vi "New ThingeverseIO Descriptor.vi"(11 "ThingiverseIO Descriptor":T2) -> (3 "Descriptor":string)   [LabVIEW 2015]
uses:
  ThingiverseIO Descriptor.ctl
  ThingerseIO Type.ctl
panel:
  in  "ThingerseIO Type":T1
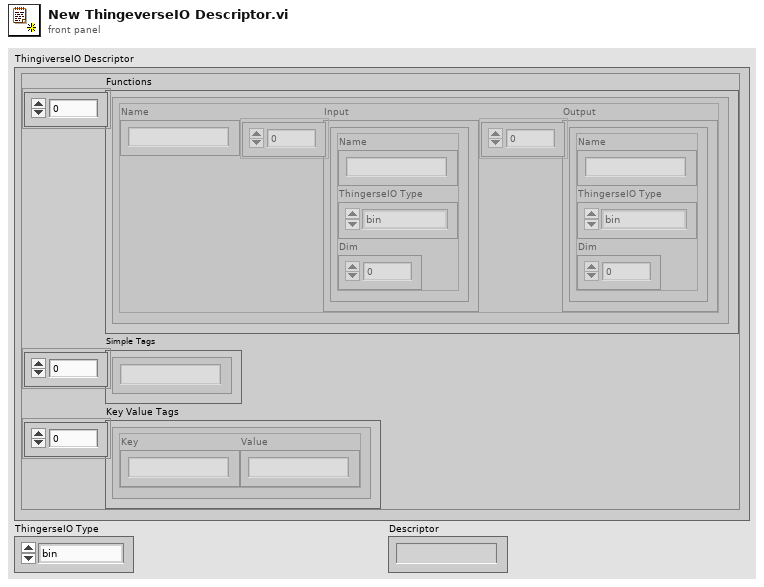
[diagram p1: front panel]
types:
  T1 = typedef "ThingerseIO Type.ctl" = enum16{"bin", "string", "Int", "float", "bool"}
  T2 = typedef "ThingiverseIO Descriptor.ctl" = cluster{"Functions":cluster{"Name":string, "Input":cluster{"Name":string, "ThingerseIO Type":T1, "Dim":u32}[], "Output":cluster{"Name":string, "ThingerseIO Type":T1, "Dim":u32}[]}[], "Simple Tags":string[], "Key Value Tags":cluster{"Key":string, "Value":string}[]}
  T3 = cluster{"Name":string, "Input":cluster{"Name":string, "ThingerseIO Type":T1, "Dim":u32}[], "Output":cluster{"Name":string, "ThingerseIO Type":T1, "Dim":u32}[]}[]
  T4 = cluster{"Name":string, "ThingerseIO Type":T1, "Dim":u32}[]
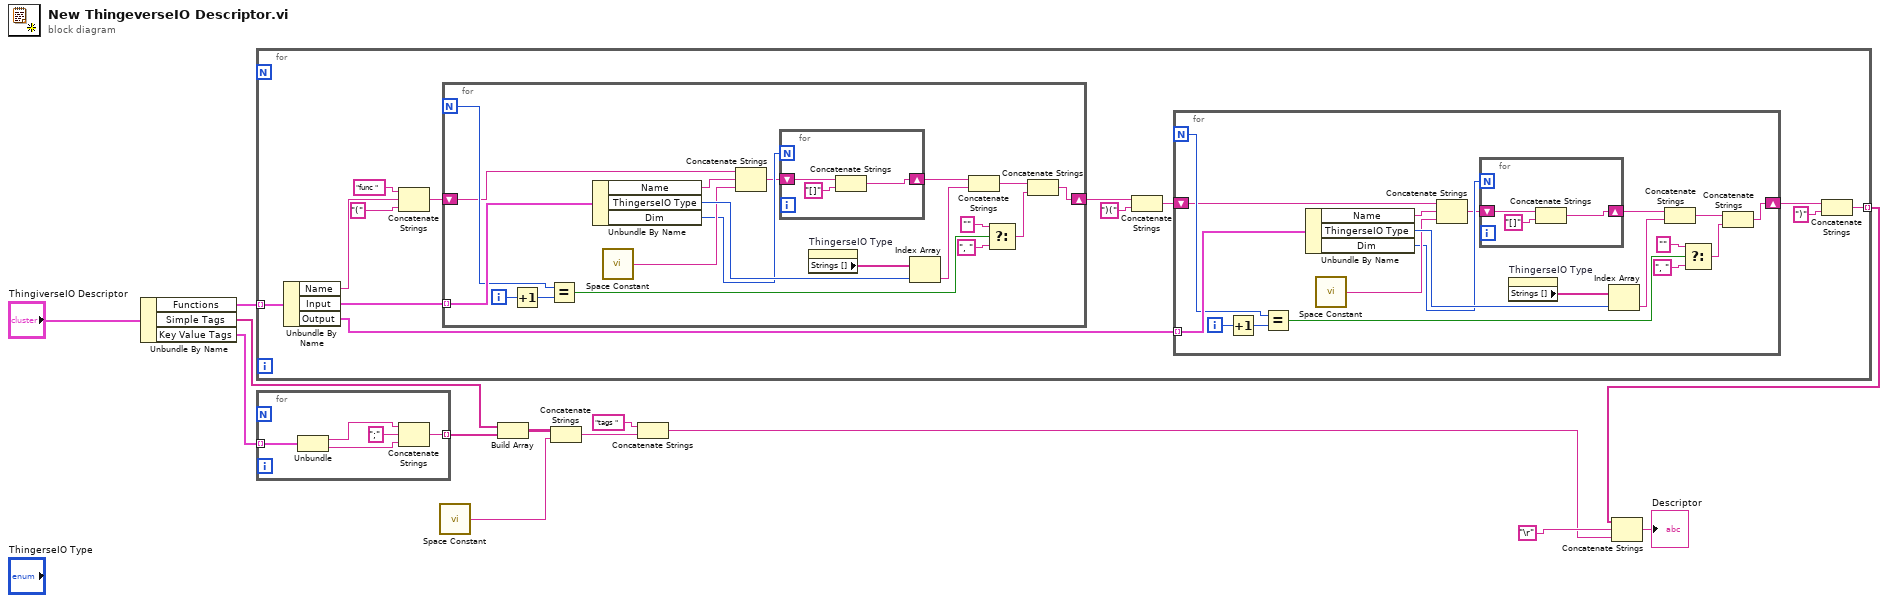
[diagram p0: block diagram]
diagram:
  n1 = Unbundle By Name("ThingiverseIO Descriptor") -> ("Functions"=w12:T3, "Simple Tags"=w10:string[], "Key Value Tags"=w11:cluster{"Key":string, "Value":string}[])
  n2 = for {
    tunnel: w12 -> [w25] mode=indexing
    tunnel: [w14] -> w4 mode=indexing
    n3 = Unbundle By Name(w25) -> ("Name"=w24:string, "Input"=w22:T4, "Output"=w18:T4)
    n4 = Concatenate Strings("func " ("string"), w24, "(" ("string")) -> (w21:string)
    n5 = for {
      N -> [w56]
      tunnel: w22 -> [w67] mode=indexing
      shift-right: [w49] -> w20
      shift-left: w21 -> [w50]
      i -> [w58]
      n6 = Increment(x=w58) -> (x+1=w57:i32)
      n7 = Equal?(x=w56, y=w57) -> (x = y?=w55:bool)
      n8 = Unbundle By Name(w67) -> ("Name"=w66:string, "ThingerseIO Type"=w64:T1, "Dim"=w62:u32)
      n9 = call <vilib>:"Space Constant.vi"() -> ("String"=w63:string)
      n10 = Concatenate Strings(w50, w66, w63) -> (w61:string)
      n11 = for {
        N: w62 -> [_]
        shift-right: [w68] -> w60
        shift-left: w61 -> [w69]
        n12 = Concatenate Strings(w69, "[]" ("string")) -> (w68:string)
      }
      n13 = property on="ThingerseIO Type" class="Enum (strict)"() -> ("Strings []"=w65:string[])  [unwired: 2 in, 2 out]
      n14 = Index Array(array=w65, index=w64) -> (element=w59:string)
      n15 = Concatenate Strings(w60, w59) -> (w52:string)
      n16 = Select(t="", s=w55, f=", " ("element")) -> (s? t:f=w51:string)
      n17 = Concatenate Strings(w52, w51) -> (w49:string)
    }
    n18 = Concatenate Strings(w20, ")(" ("string")) -> (w16:string)
    n19 = for {
      N -> [w34]
      tunnel: w18 -> [w45] mode=indexing
      shift-right: [w27] -> w15
      shift-left: w16 -> [w28]
      i -> [w36]
      n20 = Increment(x=w36) -> (x+1=w35:i32)
      n21 = Equal?(x=w34, y=w35) -> (x = y?=w33:bool)
      n22 = Unbundle By Name(w45) -> ("Name"=w44:string, "ThingerseIO Type"=w42:T1, "Dim"=w40:u32)
      n23 = call <vilib>:"Space Constant.vi"() -> ("String"=w41:string)
      n24 = Concatenate Strings(w28, w44, w41) -> (w39:string)
      n25 = for {
        N: w40 -> [_]
        shift-right: [w46] -> w38
        shift-left: w39 -> [w47]
        n26 = Concatenate Strings(w47, "[]" ("string")) -> (w46:string)
      }
      n27 = property on="ThingerseIO Type" class="Enum (strict)"() -> ("Strings []"=w43:string[])  [unwired: 2 in, 2 out]
      n28 = Index Array(array=w43, index=w42) -> (element=w37:string)
      n29 = Concatenate Strings(w38, w37) -> (w30:string)
      n30 = Select(t="", s=w33, f=", " ("element")) -> (s? t:f=w29:string)
      n31 = Concatenate Strings(w30, w29) -> (w27:string)
    }
    n32 = Concatenate Strings(w15, ")" ("string")) -> (w14:string)
  }
  n33 = for {
    tunnel: w11 -> [w74] mode=indexing
    tunnel: [w71] -> w9 mode=indexing
    n34 = Unbundle(w74) -> ("Key"=w73:string, "Value"=w72:string)
    n35 = Concatenate Strings(w73, ";" ("string"), w72) -> (w71:string)
  }
  n36 = call <vilib>:"Space Constant.vi"() -> ("String"=w7:string)
  n37 = Build Array(w10, w9) -> (w8:string[][])
  n38 = Concatenate Strings(w8, w7) -> (w6:string)
  n39 = Concatenate Strings("tags " ("string"), w6) -> (w2:string)
  n40 = Concatenate Strings(w4, "\r", w2) -> (→"Descriptor":string)
